vi "Ctor.vi"(8 "error in (no error)":errorcluster, 11 "GettingStarted in":refnum<class "GettingStarted.lvclass">) -> (0 "error out":errorcluster, 3 "GettingStarted out":refnum<class "GettingStarted.lvclass">)   [LabVIEW 2020, in "PicoG-App.lvlib" / "GettingStarted.lvclass"]
uses:
  GettingStarted.lvclass
  <vilib>/IlluminatedG/IG OOPanel/OOPanel/Panel/Panel.lvclass
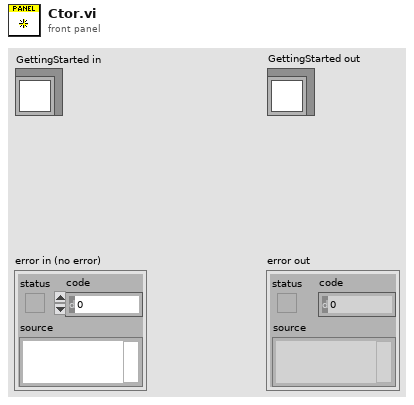
[diagram p1: front panel]
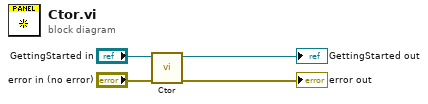
[diagram p0: block diagram]
diagram:
  n1 = call-parent "Ctor.vi"("error in (no error)"="error in (no error)", "Panel in"="GettingStarted in") -> ("error out"=→"error out":errorcluster, "Panel out"=→"GettingStarted out":refnum<class "GettingStarted.lvclass">)  [unwired: 8 in]
